vi "Load Reference.vi"(8 "error in (no error)":errorcluster, 10 "Reference":refnum<vi>, 11 "SingleStepTestV3 in":refnum<class "SingleStepTestV3.lvclass">) -> (0 "error out":errorcluster, 3 "SingleStepTestV3 out":refnum<class "SingleStepTestV3.lvclass">)   [LabVIEW 2016, in "SingleStepTestV3.lvlib" / "SingleStepTestV3.lvclass"]
doc: "The <b>Load Reference VI</b> is a dynamic dispatch VI that must be overwritten in every QControl Class and must <b>Call Parent Method</b>. This recursively loads the reference of the control to the data space for the Control Class up the inheritance hierarchy (class hierarchy). These references must be loaded in this way to use all of the built-in properties.\n\nThe reference input is the reference type needed for the control but is coerced to Generic. It should be cast back to the correct type before bundling into the class private data. The pre-casted \"Generic\" reference is wired as input to the <b>Call Parent Method</b>.\n<b> </b> <b> </b>\n©2016 Q Software Innovations, LLC (QSI)\nwritten by Quentin Alldredge\nproduced in LabVIEW 2015\n\nsupport@qsoftwareinnovations.com\nwww.qsoftwareinnovations.com\n\nAll rights reserved.\n\nRedistribution and use in source and binary forms, with or without modification, are permitted provided that the following conditions are met:\n\n * Redistributions of source code must retain the above copyright notice, this list of conditions and the following disclaimer.\n * Redistributions in binary form must reproduce the above copyright notice, this list of conditions and the following disclaimer in the documentation and/or other materials provided with the distribution.\n * Neither the name of Q Software Innovations, LLC. nor the names of its contributors may be used to endorse or promote products derived from this software without specific prior written permission.\n\nTHIS SOFTWARE IS PROVIDED BY THE COPYRIGHT HOLDERS AND CONTRIBUTORS \"AS IS\" AND ANY EXPRESS OR IMPLIED WARRANTIES, INCLUDING, BUT NOT LIMITED TO, THE IMPLIED WARRANTIES OF MERCHANTABILITY AND FITNESS FOR A PARTICULAR PURPOSE ARE DISCLAIMED. IN NO EVENT SHALL THE COPYRIGHT OWNER OR CONTRIBUTORS BE LIABLE FOR ANY DIRECT, INDIRECT, INCIDENTAL, SPECIAL, EXEMPLARY, OR CONSEQUENTIAL DAMAGES (INCLUDING, BUT NOT LIMITED TO, PROCUREMENT OF SUBSTITUTE GOODS OR SERVICES; LOSS OF USE, DATA, OR PROFITS; OR BUSINESS INTERRUPTION) HOWEVER CAUSED AND ON ANY THEORY OF LIABILITY, WHETHER IN CONTRACT, STRICT LIABILITY, OR TORT (INCLUDING NEGLIGENCE OR OTHERWISE) ARISING IN ANY WAY OUT OF THE USE OF THIS SOFTWARE, EVEN IF ADVISED OF THE POSSIBILITY OF SUCH DAMAGE."
uses:
  SingleStepTestV3.lvclass
  SingleStepTestV3.lvclass/SingleStepTestV3.ctl
  <vilib>/QSI/QControls/QControl Classes/Cluster/Cluster.lvclass
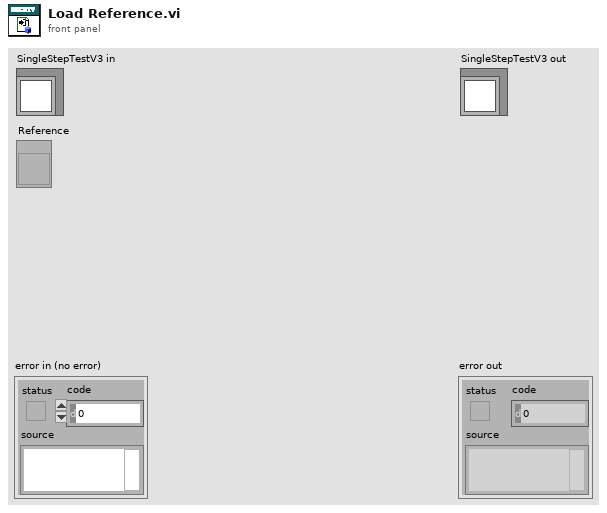
[diagram p1: front panel]
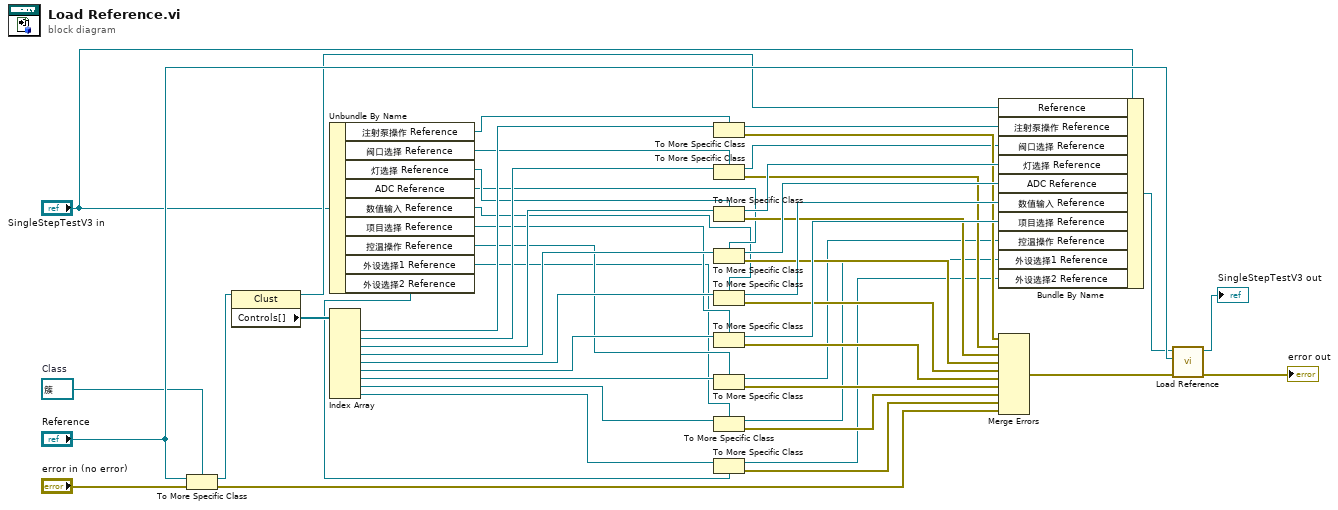
[diagram p0: block diagram]
diagram:
  w46 = refnum<vi> refnum  # Class
  n1 = To More Specific Class(target class=w46, reference="Reference", error in="error in (no error)") -> (specific class reference=w41:refnum<vi>, error out=w48:errorcluster)
  n2 = property class="Clust"(reference=w41) -> (reference out=w31:refnum<vi>, "Controls[]"=w40:refnum<vi>[])  [unwired: 1 in, 1 out]
  n3 = Unbundle By Name("SingleStepTestV3 in") -> ("注射泵操作 Reference"=w9:refnum<vi>, "阀口选择 Reference"=w8:refnum<vi>, "灯选择 Reference"=w7:refnum<vi>, "ADC Reference"=w6:refnum<vi>, "数值输入 Reference"=w5:refnum<vi>, "项目选择 Reference"=w4:refnum<vi>, "控温操作 Reference"=w3:refnum<vi>, "外设选择1 Reference"=w2:refnum<vi>, "外设选择2 Reference"=w1:refnum<vi>)
  n4 = Index Array(array=w40) -> (element #1=w39:refnum<vi>, element #2=w38:refnum<vi>, element #3=w37:refnum<vi>, element #4=w35:refnum<vi>, element #5=w30:refnum<vi>, element #6=w29:refnum<vi>, element #7=w28:refnum<vi>, element #8=w27:refnum<vi>, element #9=w26:refnum<vi>)  [unwired: 9 in]
  n5 = To More Specific Class(target class=w9, reference=w39) -> (specific class reference=w15:refnum<vi>, error out=w16:errorcluster)  [unwired: 1 in]
  n6 = To More Specific Class(target class=w8, reference=w38) -> (specific class reference=w14:refnum<vi>, error out=w17:errorcluster)  [unwired: 1 in]
  n7 = To More Specific Class(target class=w7, reference=w37) -> (specific class reference=w36:refnum<vi>, error out=w18:errorcluster)  [unwired: 1 in]
  n8 = To More Specific Class(target class=w6, reference=w35) -> (specific class reference=w34:refnum<vi>, error out=w19:errorcluster)  [unwired: 1 in]
  n9 = To More Specific Class(target class=w5, reference=w30) -> (specific class reference=w33:refnum<vi>, error out=w20:errorcluster)  [unwired: 1 in]
  n10 = To More Specific Class(target class=w4, reference=w29) -> (specific class reference=w32:refnum<vi>, error out=w21:errorcluster)  [unwired: 1 in]
  n11 = To More Specific Class(target class=w3, reference=w28) -> (specific class reference=w13:refnum<vi>, error out=w22:errorcluster)  [unwired: 1 in]
  n12 = To More Specific Class(target class=w2, reference=w27) -> (specific class reference=w12:refnum<vi>, error out=w23:errorcluster)  [unwired: 1 in]
  n13 = To More Specific Class(target class=w1, reference=w26) -> (specific class reference=w11:refnum<vi>, error out=w24:errorcluster)  [unwired: 1 in]
  n14 = Bundle By Name(cluster="SingleStepTestV3 in", "Reference"=w31, "注射泵操作 Reference"=w15, "阀口选择 Reference"=w14, "灯选择 Reference"=w36, "ADC Reference"=w34, "数值输入 Reference"=w33, "项目选择 Reference"=w32, "控温操作 Reference"=w13, "外设选择1 Reference"=w12, "外设选择2 Reference"=w11) -> (w45:refnum<class "SingleStepTestV3.lvclass">)
  n15 = Merge Errors(w16, w17, w18, w19, w20, w21, w22, w23, w24, w48) -> (w25:errorcluster)
  n16 = call-parent "Load Reference.vi"("error in (no error)"=w25, "Reference"="Reference", "Cluster in"=w45) -> ("error out"=→"error out":errorcluster, "Cluster out"=→"SingleStepTestV3 out":refnum<class "SingleStepTestV3.lvclass">)  [unwired: 7 in]
